vi "INIT.vi"(8 "error in (no error)":errorcluster, 11 "VIS-IR in":refnum<class "VIS-NIR.lvclass">) -> (0 "error out":errorcluster, 3 "VIS-IR out":refnum<class "VIS-NIR.lvclass">)   [LabVIEW 2015, in "VIS-NIR.lvclass"]
uses:
  VIS-NIR.lvclass
  GeneralFunctionality/GeneralFunctionality.lvclass/GeneralFunctionality.ctl
  Detector.lvclass/Detector.ctl
  <vilib>/addons/zeromq/socket_type.ctl
  Config/Config.lvclass
  GeneralFunctionality/GeneralFunctionality.lvclass
  Detector.lvclass
  <vilib>/addons/zeromq/zeromq.lvlib
  <vilib>/addons/zeromq/zmq_context.lvclass
  <vilib>/addons/zeromq/zmq_socket.lvclass
panel:
  in  "Dat in 10ns":u32=1
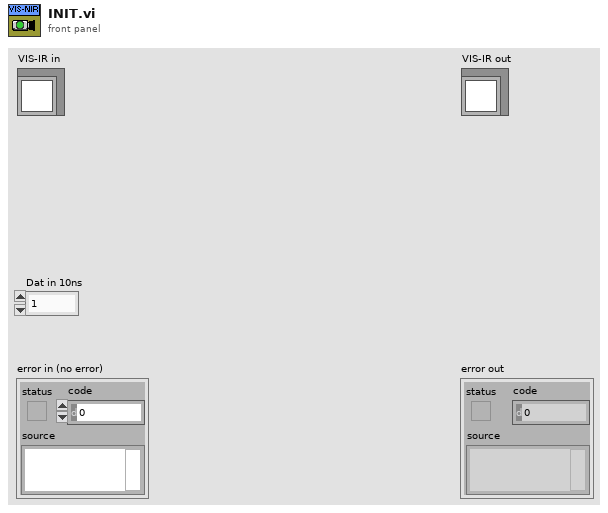
[diagram p1: front panel]
types:
  T1 = typedef "zeromq.lvlib/socket_type.ctl" = enum8{"ZMQ_PAIR", "ZMQ_PUB", "ZMQ_SUB", "ZMQ_REQ", "ZMQ_REP", "ZMQ_DEALER", "ZMQ_ROUTER", "ZMQ_PULL", "ZMQ_PUSH", "ZMQ_XPUB", "ZMQ_XSUB"}
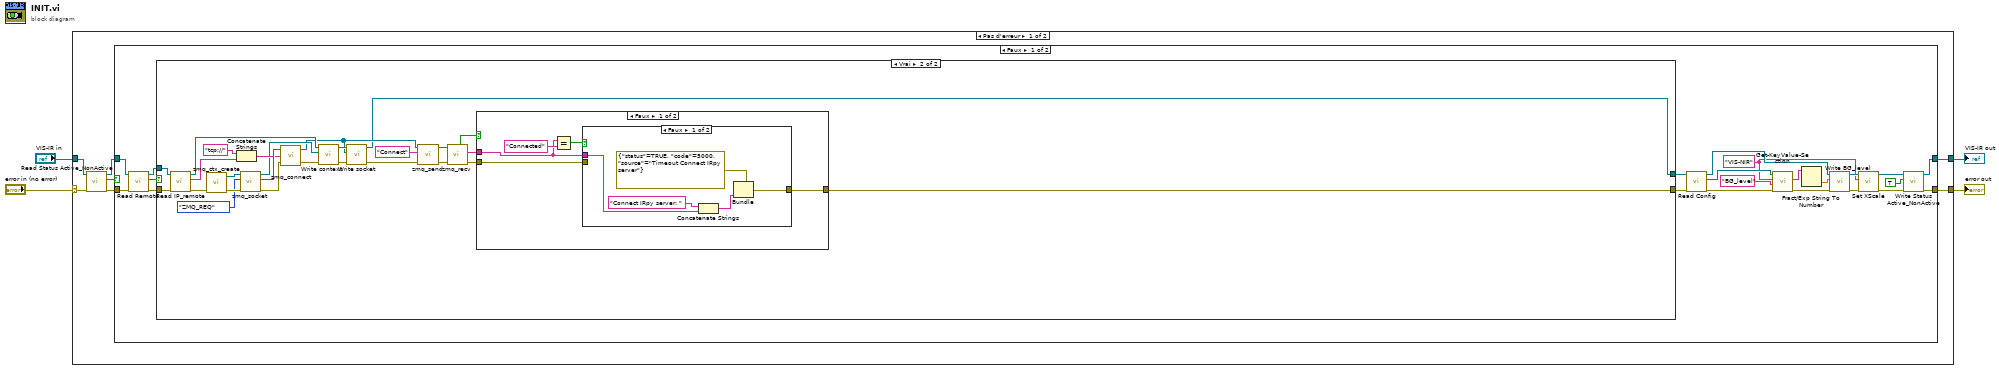
[diagram p0: block diagram]
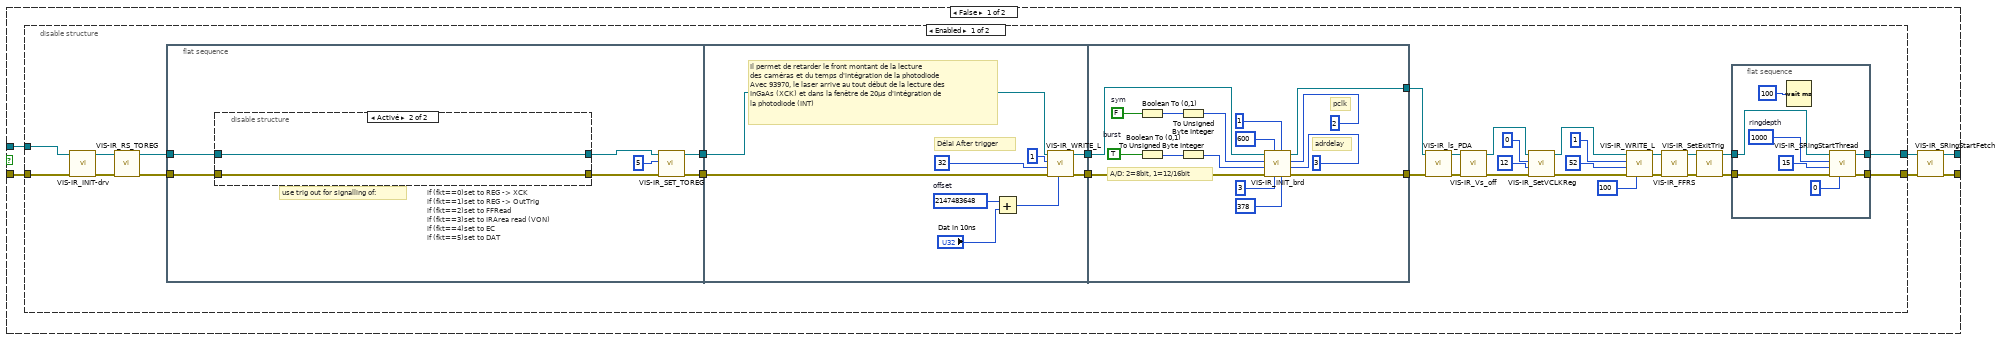
[diagram p2: hidden frame]
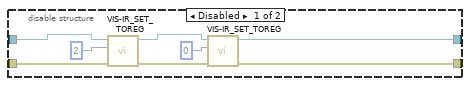
[diagram p3: hidden frame]
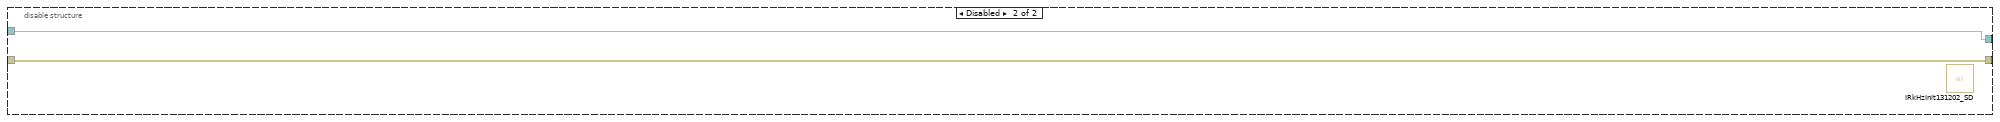
[diagram p4: hidden frame]
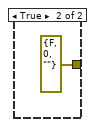
[diagram p5: hidden frame]
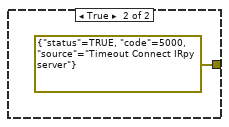
[diagram p6: hidden frame]
diagram:
  n1 = case shown="Pas d'erreur" "error in (no error)" {
    selector: "error in (no error)" -> [w8 w164]
    tunnel: "VIS-IR in" -> [w9 w163]
    tunnel: [w11 w164] -> w2
    tunnel: [w10 w163] -> w1
    frame No Error {
      n2 = call "Read Status Active_NonActive.vi"("error in (no error)"=w8, "GeneralFunctionality in"=w9) -> ("error out"=w7:errorcluster, "Status Active/NonActive"=w5:bool, "GeneralFunctionality out"=w6:refnum<class "VIS-NIR.lvclass">)  [unwired: 7 in]
      n3 = case shown="Faux" w5 {
        tunnel: [w28 w162] -> w11
        tunnel: [w27 w161] -> w10
        tunnel: w7 -> [w31 w162]
        tunnel: w6 -> [w33 w161]
        frame False {
          w12 = "VIS-NIR" ("Section")
          n4 = call "Read Remote.vi"("error in (no error)"=w31, "Detector in"=w33) -> ("error out"=w30:errorcluster, "Remote"=w29:bool, "Detector out"=w32:refnum<class "VIS-NIR.lvclass">)  [unwired: 7 in]
          n5 = case shown="Vrai" w29 {
            tunnel: [w36 w124] -> w14
            tunnel: [w37 w123] -> w16
            tunnel: w32 -> [w35 w147]
            tunnel: w30 -> [w34 w148]
            frame False {
              n6 = disable-structure shown="Enabled" {
                disable-tunnel: [w47 w122] -> w39
                disable-tunnel: [w46 w121] -> w38
                disable-tunnel: w35 -> [w41 w122]
                disable-tunnel: w34 -> [w40 w121]
                frame Enabled {
                  n7 = call "VIS-IR_INIT-drv.vi"("error in (no error)"=w40, "VIS-IR in"=w41) -> ("error out"=w45:errorcluster, "VIS-IR out"=w43:refnum<class "VIS-NIR.lvclass">)  [unwired: 8 in]
                  n8 = call "VIS-IR_RS_TOREG.vi"("error in (no error)"=w45, "VIS-IR in"=w43) -> ("error out"=w44:errorcluster, "VIS-IR out"=w42:refnum<class "VIS-NIR.lvclass">)  [unwired: 8 in]
                  n9 = flat-sequence {
                    tunnel: [w84] -> w70
                    tunnel: [w83] -> w69
                    tunnel: w42 -> [w82]
                    tunnel: w44 -> [w79]
                    tunnel: w70 -> [w104]
                    tunnel: w69 -> [w103]
                    tunnel: [w97] -> w68
                    tunnel: [w96] -> w67
                    tunnel: w68 -> [w120]
                    tunnel: w67 -> [w119]
                    tunnel: [w106] -> w66
                    tunnel: [w105] -> w65
                    frame #0 {
                      # "use trig out for signalling of:"
                      # "if (fkt==0)set to REG -> XCK\nif (fkt==1)set to REG -> OutTrig\nif (fkt==2)set to FFRead\nif (fkt==3)set to IRArea read (VON)\nif (fkt==4)set to EC\nif (fkt==5)set to DAT"
                      n10 = disable-structure shown="Activé" {
                        disable-tunnel: w82 -> [w93 w95]
                        disable-tunnel: [w91 w95] -> w81
                        disable-tunnel: [w90 w94] -> w80
                        disable-tunnel: w79 -> [w88 w94]
                        frame Disabled {
                          n11 = call "VIS-IR_SET_TOREG.vi"("error in (no error)"=w88, "fkt"=u8 2, "VIS-IR in"=w93) -> ("error out"=w89:errorcluster, "VIS-IR out"=w92:refnum<class "VIS-NIR.lvclass">)  [unwired: 7 in]
                          n12 = call "VIS-IR_SET_TOREG.vi"("error in (no error)"=w89, "fkt"=u8 0, "VIS-IR in"=w92) -> ("error out"=w90:errorcluster, "VIS-IR out"=w91:refnum<class "VIS-NIR.lvclass">)  [unwired: 7 in]
                        }
                        frame Enabled {
                        }
                      }
                      n13 = call "VIS-IR_SET_TOREG.vi"("error in (no error)"=w80, "fkt"=u8 5, "VIS-IR in"=w81) -> ("error out"=w83:errorcluster, "VIS-IR out"=w84:refnum<class "VIS-NIR.lvclass">)  [unwired: 7 in]
                    }
                    frame #1 {
                      w99 = u32 2147483648  # offset
                      # "Il permet de retarder le front montant de la lecture \ndes caméras et du temps d'intégration de la photodiode\nAvec 93970, le laser arrive au tout début de la lecture des\nInGaAs (XCK) et dans la fenêtre de 20µs d'intégration de \nla photodiode (INT)"
                      # "Délai After trigger"
                      n14 = Add(x=w99, y="Dat in 10ns") -> (x+y=w98:u32)
                      n15 = call "VIS-IR_WRITE_L.vi"("val"=w98, "error in (no error)"=w103, "offset"=u32 32, "drv"=u32 1, "VIS-IR in"=w104) -> ("error out"=w97:errorcluster, "VIS-IR out"=w96:refnum<class "VIS-NIR.lvclass">)  [unwired: 5 in]
                    }
                    frame #2 {
                      w116 = TRUE  # burst
                      w115 = FALSE  # sym
                      # "adrdelay"
                      # "pclk"
                      # "A/D: 2=8bit, 1=12/16bit"
                      n16 = Boolean To (0,1)(Boolean=w115) -> (0, 1=w117:i16)
                      n17 = Boolean To (0,1)(Boolean=w116) -> (0, 1=w118:i16)
                      n18 = To Unsigned Byte Integer(number=w117) -> (unsigned 8bit integer=w114:u8)
                      n19 = To Unsigned Byte Integer(number=w118) -> (unsigned 8bit integer=w107:u8)
                      n20 = call "VIS-IR_INIT_brd.vi"("AdrDelay"=u32 3, "pclk"=u32 2, "PPortAddress"=u32 378, "flag816"=u32 1, "waits"=u32 3, "pixel"=u32 600, "error in (no error)"=w120, "burst"=w107, "sym"=w114, "VIS-IR in"=w119) -> ("error out"=w105:errorcluster, "VIS-IR out"=w106:refnum<class "VIS-NIR.lvclass">)
                    }
                  }
                  n21 = call "VIS-IR_ls_PDA.vi"("error in (no error)"=w65, "VIS-IR in"=w66) -> ("error out"=w64:errorcluster, "VIS-IR out"=w63:refnum<class "VIS-NIR.lvclass">)  [unwired: 8 in]
                  n22 = call "VIS-IR_Vs_off.vi"("error in (no error)"=w64, "VIS-IR in"=w63) -> ("error out"=w61:errorcluster, "VIS-IR out"=w62:refnum<class "VIS-NIR.lvclass">)  [unwired: 8 in]
                  n23 = call "VIS-IR_SetVCLKReg.vi"("error in (no error)"=w61, "vfreq"=u8 12, "lines"=u32 0, "VIS-IR in"=w62) -> ("error out"=w57:errorcluster, "VIS-IR out"=w58:refnum<class "VIS-NIR.lvclass">)  [unwired: 6 in]
                  n24 = call "VIS-IR_WRITE_L.vi"("val"=u32 100, "error in (no error)"=w57, "offset"=u32 52, "drv"=u32 1, "VIS-IR in"=w58) -> ("error out"=w52:errorcluster, "VIS-IR out"=w53:refnum<class "VIS-NIR.lvclass">)  [unwired: 5 in]
                  n25 = call "VIS-IR_FFRS.vi"("error in (no error)"=w52, "VIS-IR in"=w53) -> ("error out"=w50:errorcluster, "VIS-IR out"=w51:refnum<class "VIS-NIR.lvclass">)  [unwired: 8 in]
                  n26 = call "VIS-IR_SetExitTrig.vi"("error in (no error)"=w50, "VIS-IR in"=w51) -> ("error out"=w48:errorcluster, "VIS-IR out"=w49:refnum<class "VIS-NIR.lvclass">)  [unwired: 8 in]
                  n27 = flat-sequence {
                    tunnel: [w78] -> w47
                    tunnel: [w77] -> w46
                    tunnel: w49 -> [w75]
                    tunnel: w48 -> [w74]
                    frame #0 {
                      w76 = u32 1000  # ringdepth
                      n28 = Wait (ms)(milliseconds to wait=u32 100) -> ()  [unwired: 1 out]
                      n29 = call "VIS-IR_SRingStartThread.vi"("releasems"=i16 0, "error in (no error)"=w74, "threadp"=u32 15, "ringdepth"=w76, "VIS-IR in"=w75) -> ("error out"=w77:errorcluster, "VIS-IR out"=w78:refnum<class "VIS-NIR.lvclass">)  [unwired: 5 in]
                    }
                  }
                }
                frame Disabled {
                  n30 = call "IRkHzInit131202_SD.vi"() -> ()  [unwired: 1 in]
                }
              }
              n31 = call "VIS-IR_SRingStartFetch.vi"("error in (no error)"=w38, "VIS-IR in"=w39) -> ("error out"=w36:errorcluster, "VIS-IR out"=w37:refnum<class "VIS-NIR.lvclass">)  [unwired: 8 in]
            }
            frame True {
              n32 = call "Read IP_remote.vi"("error in (no error)"=w148, "Detector in"=w147) -> ("error out"=w141:errorcluster, "IP_remote"=w139:string, "Detector out"=w134:refnum<class "VIS-NIR.lvclass">)  [unwired: 7 in]
              n33 = call <vilib>:"zmq_ctx_create.vi"("error in"=w141) -> ("error out"=w145:errorcluster, "context out"=w146:refnum<class "zmq_context.lvclass">)  [unwired: 3 in]
              n34 = Concatenate Strings("tcp://" ("endpoint"), w139) -> (w138:string)
              n35 = call <vilib>:"zmq_socket.vi"("error in"=w145, "socket type"=socket_type."ZMQ_REQ", "context in"=w146) -> ("error out"=w144:errorcluster, "socket out"=w143:refnum<class "zmq_socket.lvclass">, "context out"=w136:refnum<class "zmq_context.lvclass">)  [unwired: 2 in]
              n36 = call <vilib>:"zmq_connect.vi"("error in"=w144, "endpoint"=w138, "socket in"=w143) -> ("error out"=w137:errorcluster, "socket out"=w130:refnum<class "zmq_socket.lvclass">)  [unwired: 1 in]
              n37 = call "Write context.vi"("error in (no error)"=w137, "zeromq.lvlib:ZeroMQ Context"=w136, "Detector in"=w134) -> ("error out"=w133:errorcluster, "Detector out"=w135:refnum<class "VIS-NIR.lvclass">)  [unwired: 7 in]
              n38 = call "Write socket.vi"("error in (no error)"=w133, "zeromq.lvlib:ZeroMQ Socket"=w130, "Detector in"=w135) -> ("error out"=w131:errorcluster, "Detector out"=w123:refnum<class "VIS-NIR.lvclass">)  [unwired: 7 in]
              n39 = call <vilib>:"zmq_send.vi"("error in"=w131, "data"="Connect", "socket in"=w130) -> ("error out"=w128:errorcluster, "socket out"=w129:refnum<class "zmq_socket.lvclass">)  [unwired: 4 in]
              n40 = call <vilib>:"zmq_recv.vi"("error in"=w128, "socket in"=w129) -> ("error out"=w126:errorcluster, "data"=w125:string, "timeout?"=w127:bool)  [unwired: 3 in, 2 out]
              n41 = case shown="Faux" w127 {
                tunnel: w126 -> [w150 _]
                tunnel: [w151 errorcluster {"status"=TRUE, "code"=5000, "source"="Timeout Connect IRpy server"} ("error out")] -> w124
                tunnel: w125 -> [w149 _]
                frame False {
                  n42 = Equal?(x=w149, y="Connected") -> (x = y?=w152:bool)
                  n43 = case shown="Faux" w152 {
                    tunnel: [w154 errorcluster {"status"=FALSE, "code"=0, "source"=""} ("error out")] -> w151
                    tunnel: w150 -> [_ _]
                    tunnel: w149 -> [w156 _]
                    frame False {
                      n44 = Concatenate Strings("Connect IRpy server: ", w156) -> (w155:string)
                      n45 = Bundle(cluster=errorcluster {"status"=TRUE, "code"=5000, "source"="Timeout Connect IRpy server"} ("error out"), "source"=w155) -> (w154:errorcluster)  [unwired: 2 in]
                    }
                    frame True {
                    }
                  }
                }
                frame True {
                }
              }
            }
          }
          n46 = call "Read Config.vi"("error in (no error)"=w14, "GeneralFunctionality en entrée"=w16) -> ("error out"=w19:errorcluster, "Config.lvclass"=w18:refnum<class "Config.lvclass">, "GeneralFunctionality en sortie"=w17:refnum<class "VIS-NIR.lvclass">)  [unwired: 7 in]
          n47 = call-dynamic "Get-KeyValue-Section.vi"("error in (no error)"=w19, "Key"="BG_level", "Section"=w12, "Config in"=w18) -> ("error out"=w23:errorcluster, "Value"=w21:string)  [unwired: 5 in, 1 out]
          n48 = Fract/Exp String To Number(string=w21) -> (number=w20:dbl)  [unwired: 3 in, 1 out]
          n49 = call-dynamic "Write BG_level.vi"("error in (no error)"=w23, "BG_level"=w20, "Detector in"=w17) -> ("error out"=w13:errorcluster, "Detector out"=w15:refnum<class "VIS-NIR.lvclass">)  [unwired: 7 in]
          n50 = call "Set XScale.vi"("error in (no error)"=w13, "Section"=w12, "Detector en entrée"=w15) -> ("error out"=w24:errorcluster, "Detector en sortie"=w25:refnum<class "VIS-NIR.lvclass">)  [unwired: 7 in]
          n51 = call "Write Status Active_NonActive.vi"("error in (no error)"=w24, "Status Active/NonActive"=TRUE, "GeneralFunctionality in"=w25) -> ("error out"=w28:errorcluster, "GeneralFunctionality out"=w27:refnum<class "VIS-NIR.lvclass">)  [unwired: 7 in]
        }
        frame True {
        }
      }
    }
    frame Error {
    }
  }
  "error out" <- w2
  "VIS-IR out" <- w1
